vi "NewAutoListProcessor.vi"(11 "AutoList":T1[](array[typedef])) -> ()   [LabVIEW 2023]
uses:
  NewAutoStepTypedef.ctl
  NewAutoStepTypeEnum.ctl
  Elevator/ElevatorSetpointEnum.ctl
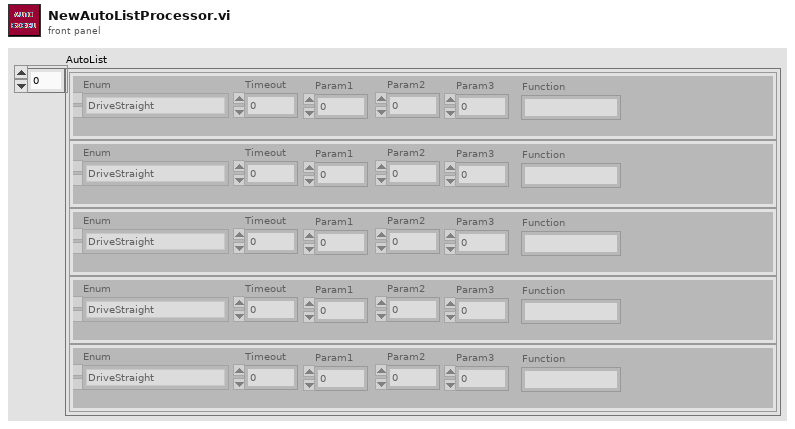
[diagram p1: front panel]
types:
  T1 = typedef "NewAutoStepTypedef.ctl" = cluster{"Enum":T2, "Timeout":dbl, "Param1":dbl, "Param2":dbl, "Param3":dbl, "Function":string}
  T2 = typedef "NewAutoStepTypeEnum.ctl" = enum16{"DriveStraight", "DriveTurn", "FollowAbsoluteTrajectory", "FollowRelativeTrajectory", "AutoWait", "ElevToRest", "ElevToFloor", "ElevToSource", "ElevToL1", "ElevToL2", "ElevToL3", "ElevToL4", "ElevToAlgae1", "ElevToAlgae2", "ElevToBarge", "ElevCancel", "IntakeCoral", "IntakeAlgae", "IntakeDepositCoral", "IntakeDepositAlgae", "IntakeCancel", "ElevRestWait", "ElevFloorWait", "ElevSourceWait", "ElevL1Wait", "ElevL2Wait", "ElevAlgae1Wait", "ElevL3Wait", "ElevAlgae2Wait", "ElevL4Wait", "ElevBargeWait"}
  T3 = typedef "ElevatorSetpointEnum.ctl" = enum16{"Floor", "Rest", "Source", "L1", "L2", "Algae1", "L3", "Algae2", "L4", "Barge"}
  T4 = typedef "Trajectory_Library.lvlib/TRAJECTORY.ctl" = cluster{"TotalTImeSecs":dbl, "States":T5[]}
  T5 = typedef "Trajectory_Library.lvlib/TRAJ_STATE.ctl" = cluster{"TimeSeconds":dbl, "Velocity":dbl, "Acceleration":dbl, "POSE":T6, "Curvature":dbl}
  T6 = typedef "Trajectory_Library.lvlib/POSE2D.ctl" = cluster{"TRANSLATION":T7, "ROTATION":T8}
  T7 = typedef "Trajectory_Library.lvlib/TRANSLATION2D.ctl" = cluster{"X":dbl, "Y":dbl}
  T8 = typedef "Trajectory_Library.lvlib/ROTATION2D.ctl" = cluster{"VALUE":dbl, "COS":dbl, "SIN":dbl}
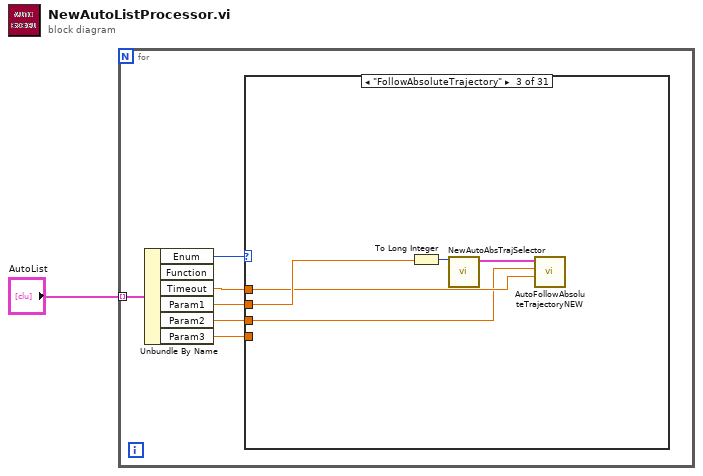
[diagram p0: block diagram]
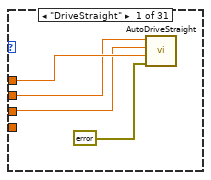
[diagram p2: hidden frame]
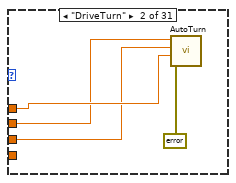
[diagram p3: hidden frame]
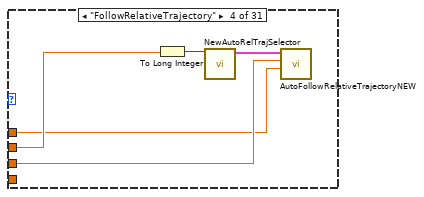
[diagram p4: hidden frame]
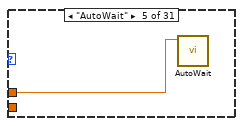
[diagram p5: hidden frame]
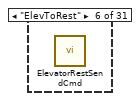
[diagram p6: hidden frame]
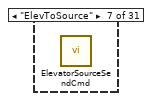
[diagram p7: hidden frame]
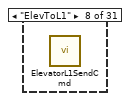
[diagram p8: hidden frame]
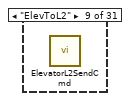
[diagram p9: hidden frame]
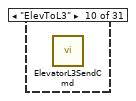
[diagram p10: hidden frame]
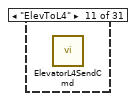
[diagram p11: hidden frame]
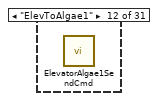
[diagram p12: hidden frame]
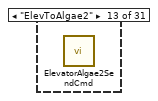
[diagram p13: hidden frame]
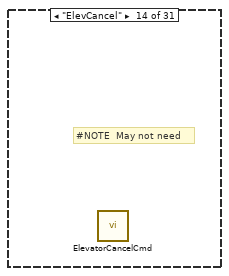
[diagram p14: hidden frame]
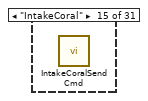
[diagram p15: hidden frame]
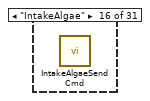
[diagram p16: hidden frame]
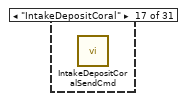
[diagram p17: hidden frame]
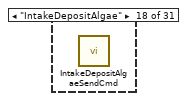
[diagram p18: hidden frame]
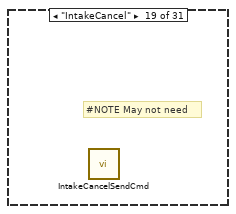
[diagram p19: hidden frame]
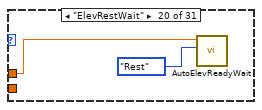
[diagram p20: hidden frame]
diagram:
  n1 = for {
    tunnel: "AutoList" -> [w7] mode=indexing
    n2 = Unbundle By Name(w7) -> ("Enum"=w6:T2, "Timeout"=w5:dbl, "Param1"=w4:dbl, "Param2"=w2:dbl, "Param3"=w3:dbl)  [unwired: 1 out]
    n3 = case shown="\"FollowAbsoluteTrajectory\"" w6 {
      tunnel: w5 -> [w11 w15 w17 w21 w26 _ _ _ _ _ _ _ _ _ _ _ _ _ _ w27 w29 w31 w33 w35 w37 w39 w41 _ _ w43 w46]
      tunnel: w4 -> [w10 w14 w18 w23 _ _ _ _ _ _ _ _ _ _ _ _ _ _ _ _ _ _ _ _ _ _ _ _ _ _ _]
      tunnel: w3 -> [_ _ _ _ _ _ _ _ _ _ _ _ _ _ _ _ _ _ _ _ _ _ _ _ _ _ _ _ _ _ _]
      tunnel: w2 -> [w9 w13 w16 w22 _ _ _ _ _ _ _ _ _ _ _ _ _ _ _ _ _ _ _ _ _ _ _ _ _ _ _]
      frame "DriveStraight" {
        n4 = call "AutoDriveStraight.vi"("error in (no error)"=errorcluster {"status"=FALSE, "code"=0, "source"=""}, "TimeOut (s)"=w11, "MaxSpeed (ft/s)"=w9, "Dist (ft)"=w10) -> ()  [unwired: 7 in, 1 out]
      }
      frame "DriveTurn" {
        n5 = call "AutoTurn.vi"("error in (no error)"=errorcluster {"status"=FALSE, "code"=0, "source"=""}, "TimeOut (s)"=w15, "MaxSpeed (ft/s)"=w13, "degrees"=w14) -> ()  [unwired: 7 in, 1 out]
      }
      frame "FollowAbsoluteTrajectory" {
        n6 = To Long Integer(number=w18) -> (32bit integer=w20:i32)
        n7 = call "NewAutoAbsTrajSelector.vi"("AbsoluteTrajectoryInput"=w20) -> ("AbsoluteTrajectoryOutput"=w19:T4)  [unwired: 10 in]
        n8 = call "AutoFollowAbsoluteTrajectoryNEW.vi"("TimeOut (s)"=w17, "End Orientation"=w16, "Trajectory"=w19) -> ()  [unwired: 8 in, 1 out]
      }
      frame "FollowRelativeTrajectory" {
        n9 = To Long Integer(number=w23) -> (32bit integer=w24:i32)
        n10 = call "NewAutoRelTrajSelector.vi"("RelativeTrajectoryInput"=w24) -> ("RelativeTrajectoryOutput"=w25:T4)  [unwired: 10 in]
        n11 = call "AutoFollowRelativeTrajectoryNEW.vi"("TimeOut (s)"=w21, "End Orientation"=w22, "Trajectory"=w25) -> ()  [unwired: 8 in, 1 out]
      }
      frame "AutoWait" {
        n12 = call "AutoWait.vi"("TimeOut (s)"=w26) -> ()  [unwired: 10 in, 1 out]
      }
      frame "ElevToRest" {
        n13 = call "ElevatorRestSendCmd.vi"() -> ()  [unwired: 11 in, 1 out]
      }
      frame "ElevToSource" {
        n14 = call "ElevatorSourceSendCmd.vi"() -> ()  [unwired: 11 in, 1 out]
      }
      frame "ElevToL1" {
        n15 = call "ElevatorL1SendCmd.vi"() -> ()  [unwired: 11 in, 1 out]
      }
      frame "ElevToL2" {
        n16 = call "ElevatorL2SendCmd.vi"() -> ()  [unwired: 11 in, 1 out]
      }
      frame "ElevToL3" {
        n17 = call "ElevatorL3SendCmd.vi"() -> ()  [unwired: 11 in, 1 out]
      }
      frame "ElevToL4" {
        n18 = call "ElevatorL4SendCmd.vi"() -> ()  [unwired: 11 in, 1 out]
      }
      frame "ElevToAlgae1" {
        n19 = call "ElevatorAlgae1SendCmd.vi"() -> ()  [unwired: 11 in, 1 out]
      }
      frame "ElevToAlgae2" {
        n20 = call "ElevatorAlgae2SendCmd.vi"() -> ()  [unwired: 11 in, 1 out]
      }
      frame "ElevCancel" {
        # "#NOTE  May not need"
        n21 = call "ElevatorCancelCmd.vi"() -> ()  [unwired: 11 in, 1 out]
      }
      frame "IntakeCoral" {
        n22 = call "IntakeCoralSendCmd.vi"() -> ()  [unwired: 11 in, 1 out]
      }
      frame "IntakeAlgae" {
        n23 = call "IntakeAlgaeSendCmd.vi"() -> ()  [unwired: 11 in, 1 out]
      }
      frame "IntakeDepositCoral" {
        n24 = call "IntakeDepositCoralSendCmd.vi"() -> ()  [unwired: 11 in, 1 out]
      }
      frame "IntakeDepositAlgae" {
        n25 = call "IntakeDepositAlgaeSendCmd.vi"() -> ()  [unwired: 11 in, 1 out]
      }
      frame "IntakeCancel" {
        # "#NOTE May not need"
        n26 = call "IntakeCancelSendCmd.vi"() -> ()  [unwired: 11 in, 1 out]
      }
      frame "ElevRestWait" {
        n27 = call "AutoElevReadyWait.vi"("ElevatorSetpoints"=ElevatorSetpointEnum."Rest", "TimeOut (s)"=w27) -> ()  [unwired: 9 in, 1 out]
      }
      frame "ElevSourceWait" {
        n28 = call "AutoElevReadyWait.vi"("ElevatorSetpoints"=ElevatorSetpointEnum."Source", "TimeOut (s)"=w29) -> ()  [unwired: 9 in, 1 out]
      }
      frame "ElevL1Wait" {
        n29 = call "AutoElevReadyWait.vi"("ElevatorSetpoints"=ElevatorSetpointEnum."L1", "TimeOut (s)"=w31) -> ()  [unwired: 9 in, 1 out]
      }
      frame "ElevL2Wait" {
        n30 = call "AutoElevReadyWait.vi"("ElevatorSetpoints"=ElevatorSetpointEnum."L2", "TimeOut (s)"=w33) -> ()  [unwired: 9 in, 1 out]
      }
      frame "ElevAlgae1Wait" {
        n31 = call "AutoElevReadyWait.vi"("ElevatorSetpoints"=ElevatorSetpointEnum."Algae1", "TimeOut (s)"=w35) -> ()  [unwired: 9 in, 1 out]
      }
      frame "ElevL3Wait" {
        n32 = call "AutoElevReadyWait.vi"("ElevatorSetpoints"=ElevatorSetpointEnum."L3", "TimeOut (s)"=w37) -> ()  [unwired: 9 in, 1 out]
      }
      frame "ElevAlgae2Wait" {
        n33 = call "AutoElevReadyWait.vi"("ElevatorSetpoints"=ElevatorSetpointEnum."Algae2", "TimeOut (s)"=w39) -> ()  [unwired: 9 in, 1 out]
      }
      frame "ElevL4Wait" {
        n34 = call "AutoElevReadyWait.vi"("ElevatorSetpoints"=ElevatorSetpointEnum."L4", "TimeOut (s)"=w41) -> ()  [unwired: 9 in, 1 out]
      }
      frame "ElevToFloor" {
        n35 = call "ElevatorFloorSendCmd.vi"() -> ()  [unwired: 11 in, 1 out]
      }
      frame "ElevToBarge" {
        n36 = call "ElevatorBargeSendCmd.vi"() -> ()  [unwired: 11 in, 1 out]
      }
      frame "ElevFloorWait" {
        n37 = call "AutoElevReadyWait.vi"("ElevatorSetpoints"=ElevatorSetpointEnum."Floor", "TimeOut (s)"=w43) -> ()  [unwired: 9 in, 1 out]
      }
      frame "ElevBargeWait" {
        n38 = call "AutoElevReadyWait.vi"("ElevatorSetpoints"=ElevatorSetpointEnum."Barge", "TimeOut (s)"=w46) -> ()  [unwired: 9 in, 1 out]
      }
    }
  }
